vi "Count_if_Subtrack_Is_Enough_for_Cost_F()(MERGE)-1.vi"(3 "[IN] Index of Earliest \nProblem Point Inside\nFisrt Part of Track":i32, 4 "[IN] Index of Problem \nPoint Inside Second Track":i32, 5 "[IN] Minimal Subtrack Length \n(Points without problems) for\nMaking Desicion":i32, 6 "[IN] Track Statuses in second\npart for track making":i16[](array[numeric])) -> (1 "[OUT] Index of Last \nPoint in Second Track":i32, 2 "[OUT] It's enough to make\nconclusion using subtrack":bool)   [LabVIEW 2013]
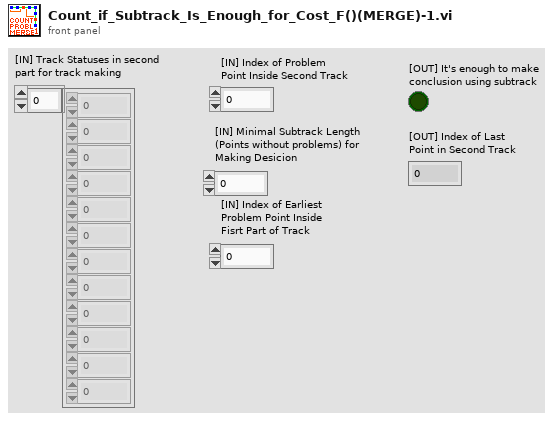
[diagram p1: front panel]
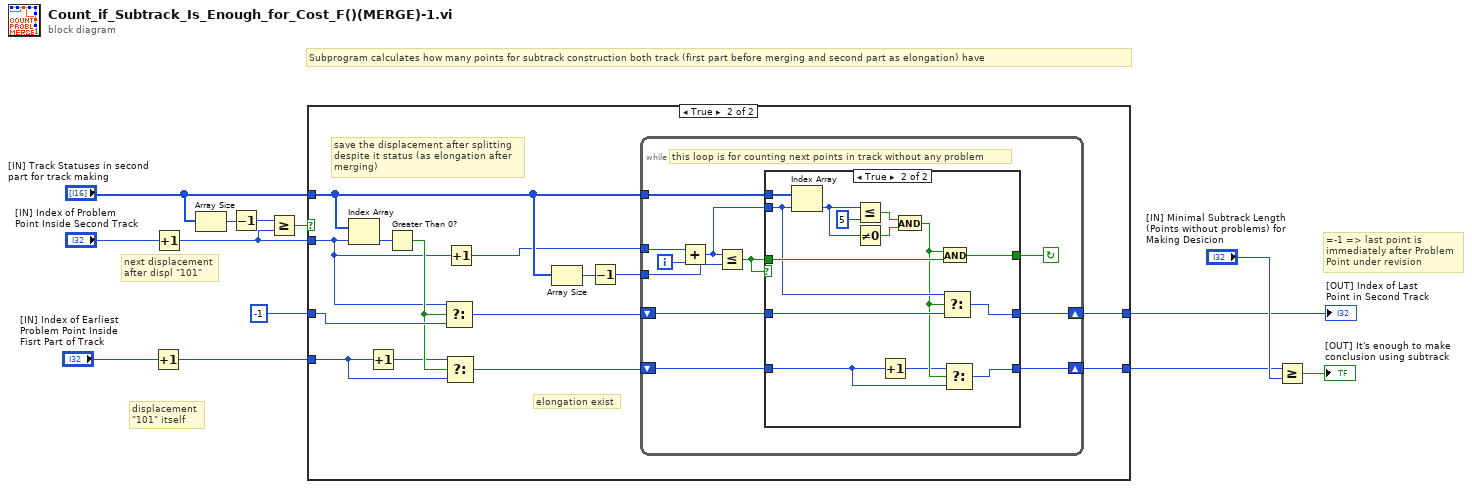
[diagram p0: block diagram]
diagram:
  # "next displacement\nafter displ \"101\""
  # "displacement \n\"101\" itself"
  # "=-1 => last point is\nimmediately after Problem \nPoint under revision"
  # "Subprogram calculates how many points for subtrack construction both track (first part before merging and second part as elongation) have"
  n1 = Increment(x="[IN] Index of Earliest \nProblem Point Inside\nFisrt Part of Track") -> (x+1=w3:i32)
  n2 = Increment(x="[IN] Index of Problem \nPoint Inside Second Track") -> (x+1=w4:i32)
  n3 = Array Size(array="[IN] Track Statuses in second\npart for track making") -> (size(s)=w8:i32)
  n4 = Decrement(x=w8) -> (x-1=w6:i32)
  n5 = Greater Or Equal?(x=w6, y=w4) -> (x >= y?=w5:bool)
  n6 = case shown="True" w5 {
    tunnel: "[IN] Track Statuses in second\npart for track making" -> [_ w25]
    tunnel: [w14 w27] -> w11
    tunnel: w4 -> [_ w17]
    tunnel: w3 -> [w15 w18]
    tunnel: [w15 w26] -> w2
    tunnel: -1 -> [w14 w23]
    frame False {
    }
    frame True {
      # "save the displacement after splitting \ndespite it status (as elongation after\nmerging)"
      # "elongation exist"
      n7 = Index Array(array=w25, index=w17) -> (element=w24:i16)
      n8 = Increment(x=w18) -> (x+1=w20:i32)
      n9 = Greater Than 0?(x=w24) -> (x > 0?=w21:bool)
      n10 = Select(t=w17, s=w21, f=w23) -> (s? t:f=w22:i32)
      n11 = Select(t=w20, s=w21, f=w18) -> (s? t:f=w19:i32)
      n12 = Increment(x=w17) -> (x+1=w16:i32)
      n13 = Array Size(array=w25) -> (size(s)=w29:i32)
      n14 = Decrement(x=w29) -> (x-1=w28:i32)
      n15 = while {
        tunnel: w28 -> [w40]
        tunnel: w16 -> [w33]
        tunnel: w25 -> [w39]
        shift-right: [w34] -> w27
        shift-left: w22 -> [w35]
        shift-right: [w30] -> w26
        shift-left: w19 -> [w31]
        i -> [w32]
        stop <- w36 continue-if-true
        # "this loop is for counting next points in track without any problem"
        n16 = Add(x=w33, y=w32) -> (x+y=w38:i32)
        n17 = Less Or Equal?(x=w38, y=w40) -> (x <= y?=w37:bool)
        n18 = case shown="True" w37 {
          tunnel: w39 -> [_ w57]
          tunnel: w38 -> [_ w48]
          tunnel: w37 -> [w43 w51]
          tunnel: [w43 w52] -> w36
          tunnel: w35 -> [w42 w49]
          tunnel: [w42 w50] -> w34
          tunnel: w31 -> [w41 w45]
          tunnel: [w41 w44] -> w30
          frame False {
            # "it's last point in subtrack"
          }
          frame True {
            n19 = Index Array(array=w57, index=w48) -> (element=w55:i16)
            n20 = Less Or Equal?(x=w55, y=i16 5) -> (x <= y?=w54:bool)
            n21 = Not Equal To 0?(x=w55) -> (x != 0?=w53:bool)
            n22 = Increment(x=w45) -> (x+1=w46:i32)
            n23 = And(x=w54, y=w53) -> (x .and. y?=w47:bool)
            n24 = And(x=w47, y=w51) -> (x .and. y?=w52:bool)
            n25 = Select(t=w48, s=w47, f=w49) -> (s? t:f=w50:i32)
            n26 = Select(t=w46, s=w47, f=w45) -> (s? t:f=w44:i32)
          }
        }
      }
    }
  }
  "[OUT] Index of Last \nPoint in Second Track" <- w11
  n27 = Greater Or Equal?(x=w2, y="[IN] Minimal Subtrack Length \n(Points without problems) for\nMaking Desicion") -> (x >= y?=→"[OUT] It's enough to make\nconclusion using subtrack":bool)
